vi "link_creation.vi"(0 "content":string, 1 "select atribute":bool, 2 "href":string, 3 "name":string, 4 "need_atribute":bool) -> (5 "result":string)   [LabVIEW 2014]
panel:
  # "href"
  # "name"
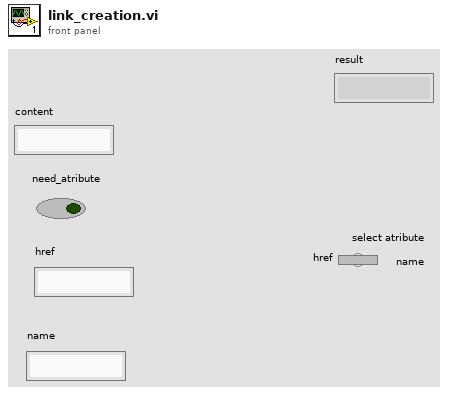
[diagram p1: front panel]
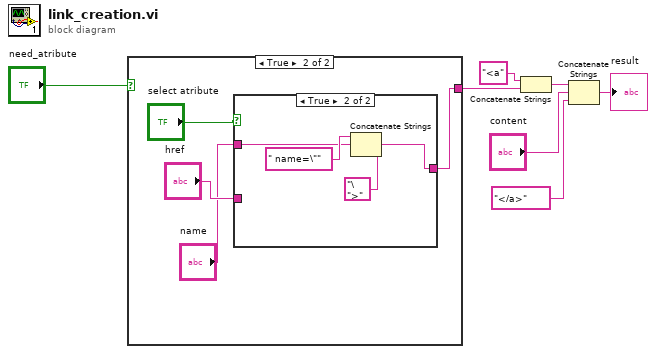
[diagram p0: block diagram]
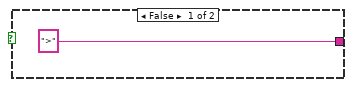
[diagram p2: hidden frame]
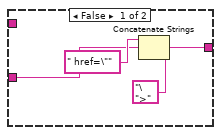
[diagram p3: hidden frame]
diagram:
  n1 = case shown="True" "need_atribute" {
    tunnel: [">" w11] -> w2
    frame False {
    }
    frame True {
      n2 = case shown="True" "select atribute" {
        tunnel: "href" -> [w15 _]
        tunnel: [w13 w17] -> w11
        tunnel: "name" -> [_ w18]
        frame False {
          n3 = Concatenate Strings(" href=\"" ("string"), w15, "\">" ("string")) -> (w13:string)
        }
        frame True {
          n4 = Concatenate Strings(" name=\"" ("string"), w18, "\">" ("string")) -> (w17:string)
        }
      }
    }
  }
  n5 = Concatenate Strings("<a" ("string"), w2) -> (w1:string)
  n6 = Concatenate Strings(w1, "content", "</a>" ("string")) -> (→"result":string)
